vi "Read Scale.vi"(9 "Knob in":refnum<class "Knob.lvclass">) -> (3 "Knob out":refnum<class "Knob.lvclass">, 4 "Scale":refnum<class "Scale.lvclass">)   [LabVIEW 2014, in "Knob.lvclass"]
uses:
  Knob.lvclass
  Scale/Scale.lvclass
  Knob.lvclass/Knob.ctl
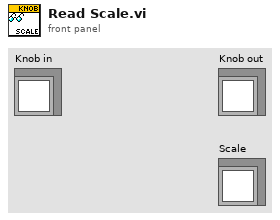
[diagram p1: front panel]
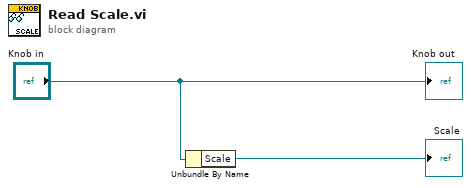
[diagram p0: block diagram]
diagram:
  n1 = Unbundle By Name("Knob in") -> ("Scale"=→"Scale":refnum<class "Scale.lvclass">)
  "Knob out" <- "Knob in"
